vi "Moments (SubVI).vi"(0 "Data":dbl[][](array[numeric]), 1 "OUT_Interp":dbl[](array[numeric])=[0.0, 0.0, 0.0, 0.0, 0.0], 2 "FE_b [N], FG [N], FA [N], Fco[N]":T6, 3 "FE [N]":dbl[](array[numeric]), 5 "V_Wind [m/s]":dbl[][](array[numeric]), 7 "Pdin [Pa], Patm [Pa], Temp [K], airflow velocity [m/s]":T3, 11 "Vehicle Parameters":T2, 12 "i, sim_running, t[s], dt[s]":T4, 13 "Rotation":T1, 14 "V(i) [m/s] NWU, latd(i) [rad], lon(i) [rad], height(i) [m]":T5) -> (8 "ang_acc":dbl[](array[numeric]))   [LabVIEW 2017]
uses:
  <vilib>/Analysis/baseanly.llb/Real A x B.vi
  <vilib>/Analysis/Matrix/Numeric/Conversions/Array To Matrix - RA.vi
  <vilib>/Analysis/Matrix/Numeric/Conversions/Array To Matrix - RA2.vi
  <vilib>/Analysis/Matrix/Numeric/Conversions/Matrix To Array - RM.vi
  <vilib>/Analysis/NI_AALBase.lvlib
  <vilib>/Analysis/Matrix/NI_Matrix.lvlib
panel:
  out "MFE_b":dbl[](array[numeric])
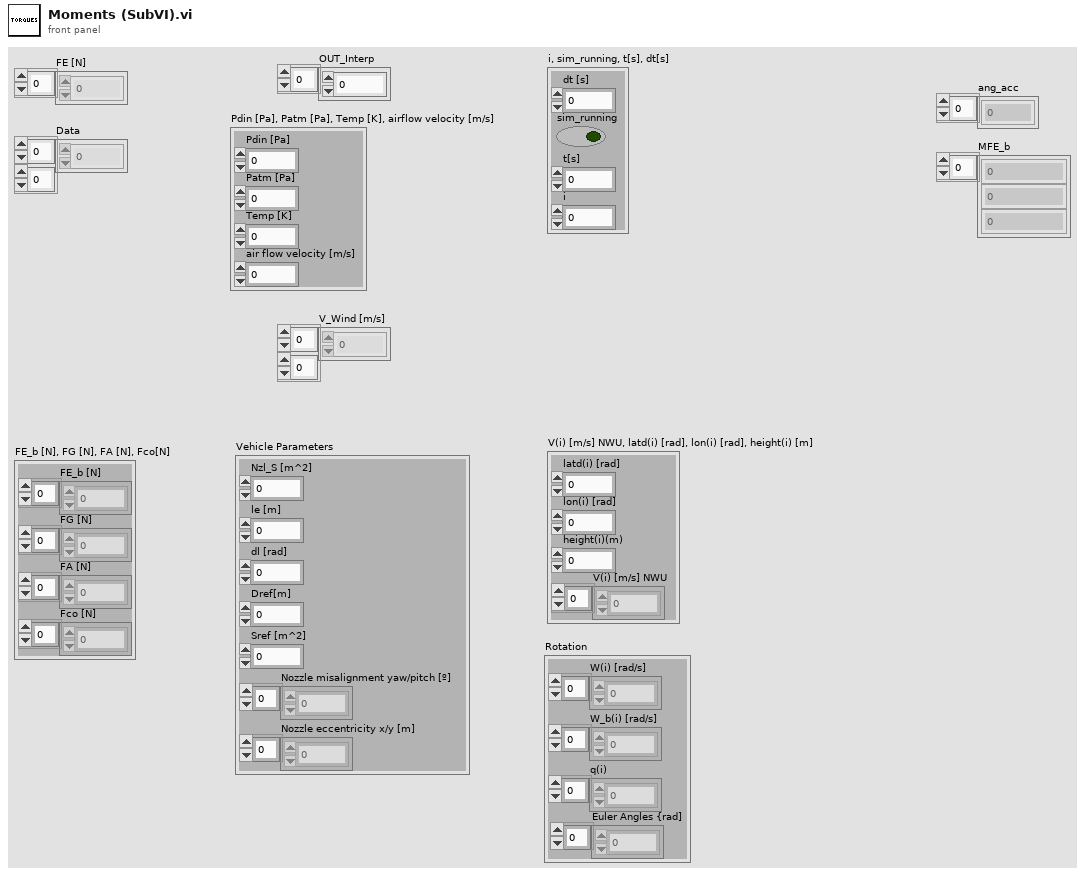
[diagram p1: front panel]
types:
  T1 = cluster{"W(i) [rad/s]":dbl[], "W_b(i) [rad/s]":dbl[], "q(i)":dbl[], "Euler Angles {rad]":dbl[]}
  T2 = cluster{"Nzl_S [m^2]":dbl, "le [m]":dbl, "dl [rad]":dbl, "Dref[m]":dbl, "Sref [m^2]":dbl, "Nozzle misalignment yaw/pitch [º]":dbl[], "Nozzle eccentricity x/y [m]":dbl[]}
  T3 = cluster{"Pdin [Pa]":dbl, "Patm [Pa]":dbl, "Temp [K]":dbl, "air flow velocity [m/s]":dbl}
  T4 = cluster{"dt [s]":dbl, "sim_running":bool, "t[s]":dbl, "i":i32}
  T5 = cluster{"latd(i) [rad]":dbl, "lon(i) [rad]":dbl, "height(i)(m)":dbl, "V(i) [m/s] NWU":dbl[]}
  T6 = cluster{"FE_b [N]":dbl[], "FG [N]":dbl[], "FA [N]":dbl[], "Fco [N]":dbl[]}
  T7 = cluster{"Mco [Nm]":dbl[], "MFE [Nm]":dbl[], "MFA [Nm]":dbl[], "MA_f [Nm]":dbl[], "MAd [Nm]":dbl[], "MAd_b":dbl[]}
  T8 = typedef "NI_Matrix.lvlib/RealMatrix.ctl" = dbl[][]
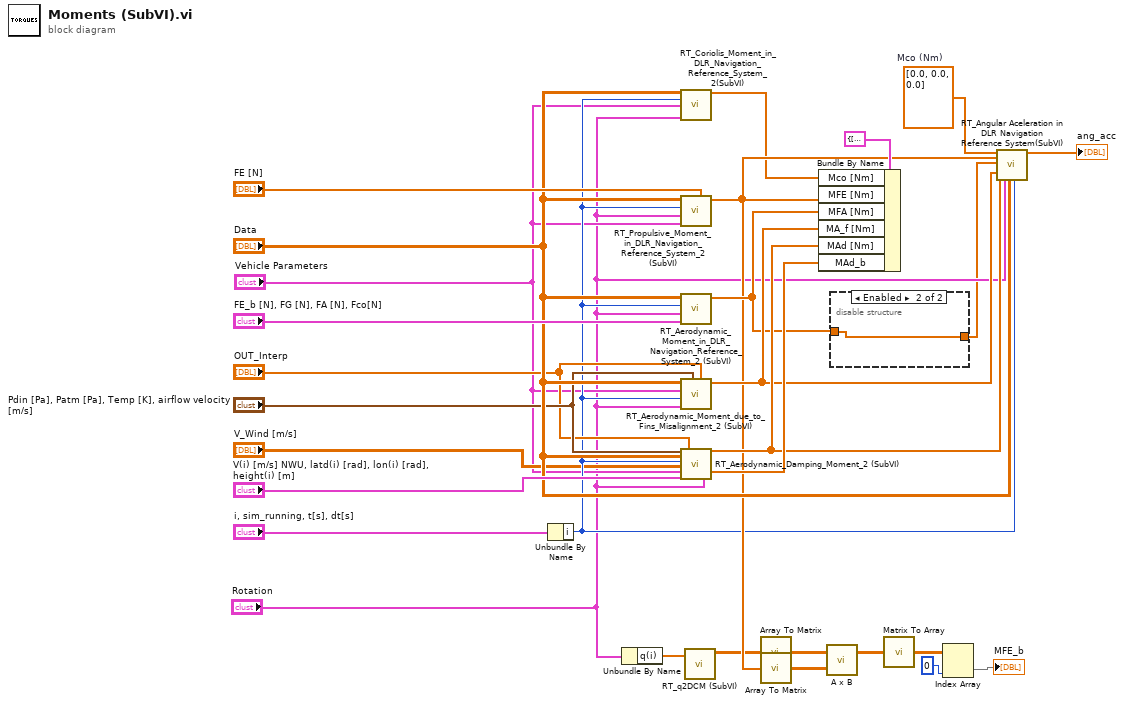
[diagram p0: block diagram]
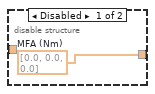
[diagram p2: hidden frame]
diagram:
  w13 = dbl[] [0.0, 0.0, 0.0]  # Mco (Nm)
  n1 = Unbundle By Name("i, sim_running, t[s], dt[s]") -> ("i"=w15:i32)
  n2 = Unbundle By Name("Rotation") -> ("q(i)"=w4:dbl[])
  n3 = call "RT_Coriolis_Moment_in_DLR_Navigation_Reference_System_2(SubVI).vi"("Data"="Data", "i"=w15, "Vehicle Parameters"="Vehicle Parameters", "Rotation"="Rotation") -> ("Mco (Nm)"=w16:dbl[])  [unwired: 11 in]
  n4 = call "RT_Propulsive_Moment_in_DLR_Navigation_Reference_System_2 (SubVI).vi"("FE"="FE [N]", "Vehicle Parameters"="Vehicle Parameters", "Rotation"="Rotation", "i"=w15, "Data"="Data") -> ("MFE (Nm)"=w17:dbl[])  [unwired: 6 in]
  n5 = call "RT_Aerodynamic_Moment_in_DLR_Navigation_Reference_System_2 (SubVI).vi"("input cluster"="FE_b [N], FG [N], FA [N], Fco[N]", "Rotation"="Rotation", "i"=w15, "Data"="Data") -> ("MFA (Nm)"=w18:dbl[])  [unwired: 7 in]
  n6 = call "RT_Aerodynamic_Moment_due_to_Fins_Misalignment_2 (SubVI).vi"("OUT_Interp"="OUT_Interp", "input cluster 2"="Pdin [Pa], Patm [Pa], Temp [K], airflow velocity [m/s]", "Rotation"="Rotation", "i"=w15, "Vehicle Parameters"="Vehicle Parameters", "Data"="Data") -> ("MA_f"=w19:dbl[])  [unwired: 5 in]
  n7 = call "RT_Aerodynamic_Damping_Moment_2 (SubVI).vi"("input cluster"="Pdin [Pa], Patm [Pa], Temp [K], airflow velocity [m/s]", "Data"="Data", "i"=w15, "V_wind [m/s]"="V_Wind [m/s]", "Vehicle Parameters"="Vehicle Parameters", "input cluster 3"="V(i) [m/s] NWU, latd(i) [rad], lon(i) [rad], height(i) [m]", "Mach coeficients"="OUT_Interp", "Rotation"="Rotation") -> ("MAd"=w20:dbl[], "MAd_b"=w21:dbl[])  [unwired: 10 in]
  n8 = call "RT_q2DCM (SubVI).vi"("Quaternion"=w4) -> ("DCM"=w3:dbl[][])  [unwired: 10 in]
  n9 = call-poly <vilib>:"Array To Matrix.vi"("Real 2D Array"=w3) -> ("Real Matrix"=w11:T8)
  n10 = call-poly <vilib>:"Array To Matrix.vi"("Real 1D Array"=w17) -> ("Real Matrix (Column Vector)"=w6:T8)
  n11 = Bundle By Name(cluster=T7 {"Mco [Nm]"=[], "MFE [Nm]"=[], "MFA [Nm]"=[], "MA_f [Nm]"=[], "MAd [Nm]"=[], "MAd_b"=[]} ("output cluster 2"), "Mco [Nm]"=w16, "MFE [Nm]"=w17, "MFA [Nm]"=w18, "MA_f [Nm]"=w19, "MAd [Nm]"=w20, "MAd_b"=w21) -> ()  [unwired: 1 out]
  n12 = call-poly <vilib>:"A x B.vi"("B"=w6, "A"=w11) -> ("A x B"=w8:T8)  [unwired: 1 out]
  n13 = disable-structure shown="Enabled" {
    disable-tunnel: w18 -> [_ w31]
    disable-tunnel: [w30 w31] -> w1
    frame Disabled {
      w30 = dbl[] [0.0, 0.0, 0.0]  # MFA (Nm)
    }
    frame Enabled {
    }
  }
  n14 = call-poly <vilib>:"Matrix To Array.vi"("Real Matrix"=w8) -> ("Real 2D Array"=w7:dbl[][])
  n15 = Index Array(array=w7, index (col)=0 ("index (row)")) -> (element=→"MFE_b":dbl[])  [unwired: 1 in]
  n16 = call "RT_Angular Aceleration in DLR Navigation Reference System(SubVI).vi"("Mco (Nm)"=w13, "MFE (Nm)"=w17, "MFA (Nm)"=w1, "MA_f [Nm]"=w19, "MAd [Nm]"=w20, "Rotation"="Rotation", "Data"="Data", "i"=w15) -> ("ang_acc"=→"ang_acc":dbl[])  [unwired: 9 in, 2 out]
